vi "Generate Physical Coordinates.vi"(9 "end":dbl=1.0 format="%0.2f", 10 "start":dbl format="%0.2f", 11 "samples":i32=128) -> (2 "output array":cluster{dbl, dbl}[](array[cluster]), 3 "Array":cluster{dbl, dbl}[][](array[cluster]))   [LabVIEW 2014]
uses:
  <vilib>/Analysis/1siggen.llb/Ramp Pattern by Samples.vi
  <vilib>/Analysis/NI_AALBase.lvlib
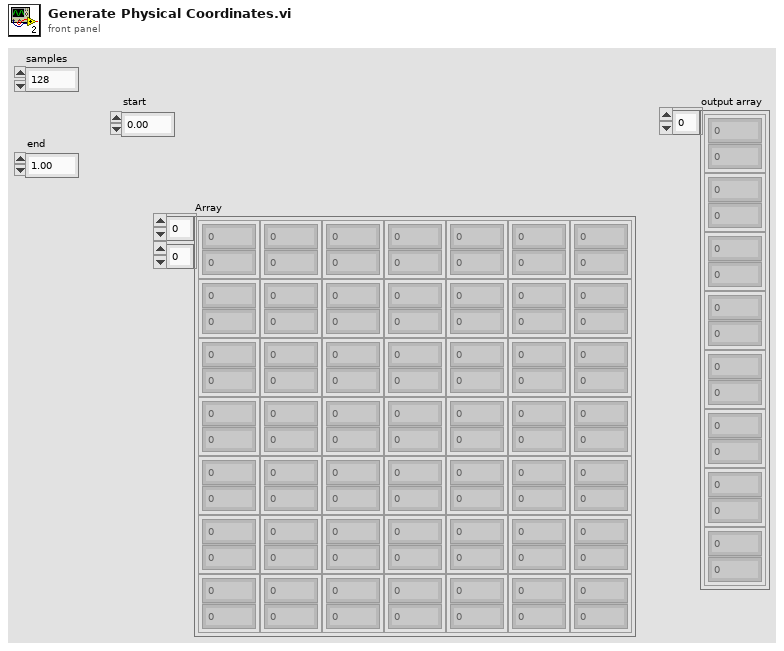
[diagram p1: front panel]
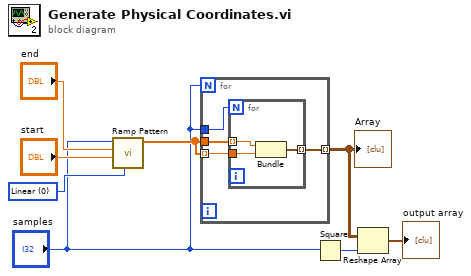
[diagram p0: block diagram]
diagram:
  w8 = u16 0 items=["Linear", "Logarithmic"] ("type")
  n1 = call-poly <vilib>:"Ramp Pattern.vi"("type"=w8, "start"="start", "end"="end", "samples"="samples") -> ("Ramp Pattern"=w5:dbl[])  [unwired: 6 in, 1 out]
  n2 = for {
    N: "samples" -> [_]
    tunnel: "samples" -> [w12]
    tunnel: w5 -> [w11]
    tunnel: w5 -> [w10] mode=indexing
    tunnel: [w9] -> w4 mode=indexing
    n3 = for {
      N: w12 -> [_]
      tunnel: w11 -> [w15] mode=indexing
      tunnel: w10 -> [w14]
      tunnel: [w13] -> w9 mode=indexing
      n4 = Bundle(w15, w14) -> (w13:cluster{dbl, dbl})  [unwired: 1 in]
    }
  }
  "Array" <- w4
  n5 = Square(x="samples") -> (x^2=w2:i32)
  n6 = Reshape Array(w4, w2) -> (→"output array":cluster{dbl, dbl}[])
